vi "MC-21C Driver_translator.vi"(4 "Step":string, 5 "Operation":enum16{"forward", "backward", "stop"}(ring), 6 "Address":u8) -> (1 "Write buffer":string)   [LabVIEW 2023]
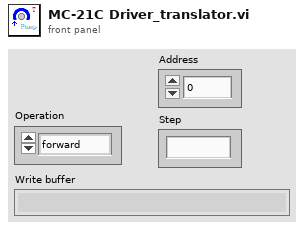
[diagram p1: front panel]
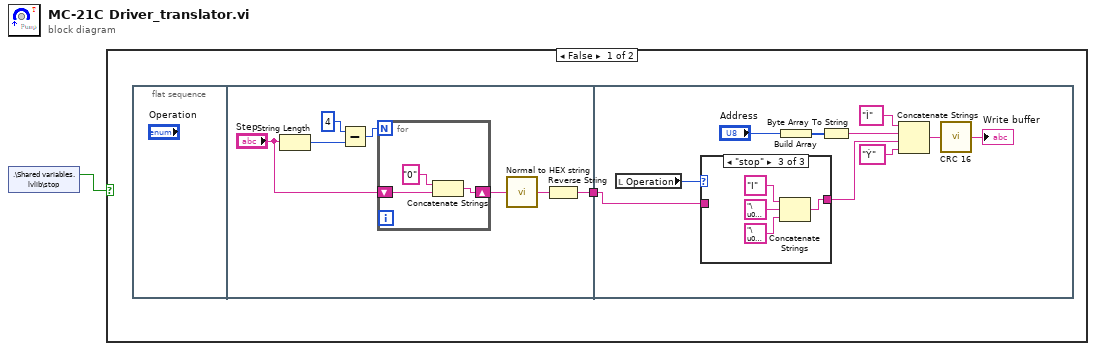
[diagram p0: block diagram]
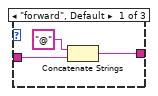
[diagram p2: hidden frame]
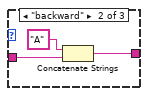
[diagram p3: hidden frame]
diagram:
  n1 = shared-variable ".\\Shared variables.lvlib\\stop"() -> (w1:bool)  [unwired: 1 in, 1 out]
  n2 = case shown="False" w1 {
    frame False {
      n3 = flat-sequence {
        tunnel: [w3] -> w2
        tunnel: w2 -> [w22]
        frame #0 {
        }
        frame #1 {
          n4 = String Length(string="Step") -> (length=w6:i32)
          n5 = Subtract(x=4, y=w6) -> (x-y=w7:i32)
          n6 = for {
            N: w7 -> [_]
            shift-right: [w10] -> w9
            shift-left: "Step" -> [w12]
            n7 = Concatenate Strings("0" ("string"), w12) -> (w10:string)
          }
          n8 = call "Normal to HEX string.vi"("input normal string"=w9) -> ("output HEX string"=w5:string)
          n9 = Reverse String(1:w5) -> (0:w3:string)
        }
        frame #2 {
          n10 = local read "Operation"() -> (w17:enum16{"forward", "backward", "stop"})
          n11 = case shown="\"stop\"" w17 {
            tunnel: w22 -> [w24 w27 _]
            tunnel: [w23 w26 w29] -> w16
            frame "forward", Default {
              n12 = Concatenate Strings("@" ("string"), w24) -> (w23:string)
            }
            frame "backward" {
              n13 = Concatenate Strings("A" ("string"), w27) -> (w26:string)
            }
            frame "stop" {
              n14 = Concatenate Strings("I" ("string"), "\u0000" ("string"), "\u0000" ("string")) -> (w29:string)
            }
          }
          n15 = Build Array("Address") -> (w20:u8[])
          n16 = Byte Array To String(unsigned byte array=w20) -> (string=w18:string)
          n17 = Concatenate Strings("Ì" ("string"), w18, w16, "Ý" ("string")) -> (w14:string)
          n18 = call "CRC 16.vi"("input HEX string"=w14) -> ("output HEX string"=→"Write buffer":string)
        }
      }
    }
    frame True {
    }
  }
